vi "Get Tasks.vi"(6 "Authorization":T2[](array[typedef]), 8 "error in (no error)":errorcluster, 11 "Project GID":string) -> (0 "error out":errorcluster, 2 "data":T1(array[cluster]))   [LabVIEW 2016]
uses:
  <vilib>/addons/_JKI.lib/REST Client/classes/REST Client/HTTP Header.ctl
  <vilib>/addons/_JKI.lib/REST Client/classes/REST Client/REST Client.lvclass
  <vilib>/addons/_JKI.lib/Serialization/JSON/JKI JSON Serialization.lvlib
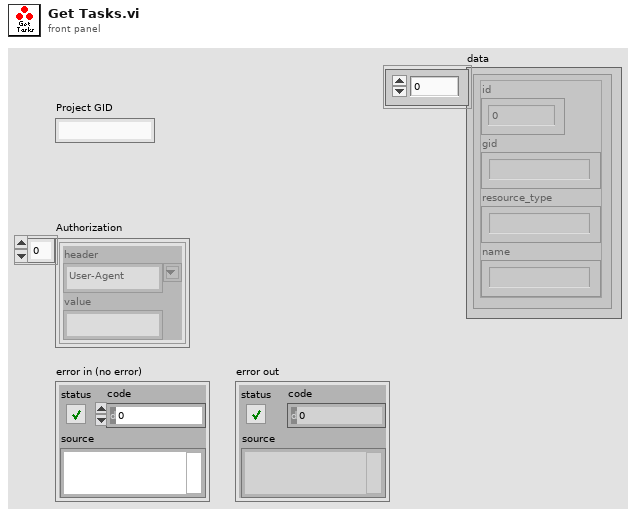
[diagram p1: front panel]
types:
  T1 = cluster{"id":i64, "gid":string, "resource_type":string, "name":string}[]
  T2 = typedef "REST Client.lvlib/REST Client.lvclass/HTTP Header.ctl" = cluster{"header":string, "value":string}
  T3 = cluster{"data":cluster{"id":i64, "gid":string, "resource_type":string, "name":string}[]}
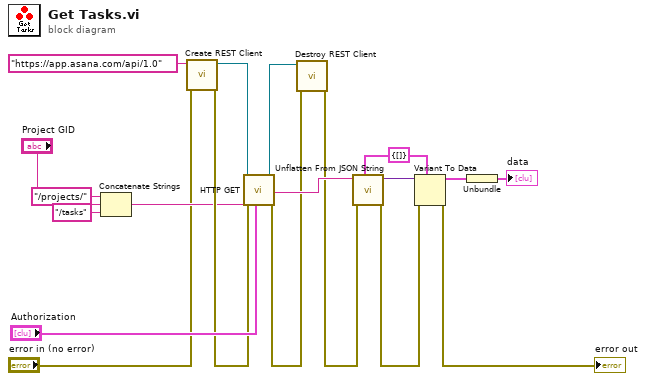
[diagram p0: block diagram]
diagram:
  w3 = T3 {"data"=[]}
  n1 = Concatenate Strings("/projects/" ("string"), "Project GID", "/tasks" ("string")) -> (w13:string)
  n2 = call <vilib>:"Create REST Client.vi"("error in (no error)"="error in (no error)", "Base URL"="https://app.asana.com/api/1.0") -> ("error out"=w16:errorcluster, "REST Client out"=w19:refnum<class "REST Client.lvclass">)  [unwired: 8 in]
  n3 = call-dynamic "HTTP GET.vi"("request specific headers"="Authorization", "error in (no error)"=w16, "Path"=w13, "REST Client in"=w19) -> ("error out"=w8:errorcluster, "Response body"=w10:string, "REST Client out"=w18:refnum<class "REST Client.lvclass">)  [unwired: 2 in, 3 out]
  n4 = call-dynamic "Destroy REST Client.vi"("error in (no error)"=w8, "REST Client in"=w18) -> ("error out"=w7:errorcluster)  [unwired: 9 in]
  n5 = call <vilib>:"Unflatten From JSON String.vi"("Type and Defaults"=w3, "error in (no error)"=w7, "JSON String"=w10) -> ("error out"=w6:errorcluster, "Variant"=w9:variant)  [unwired: 7 in]
  n6 = Variant To Data(error in=w6, type=w3, Variant=w9) -> (data=w2:T3, error out=→"error out":errorcluster)
  n7 = Unbundle(w2) -> ("data"=→"data":T1)
